vi "VelocityTorqueCurrentFOC SetControl.vi"(0 "DeviceReference":T1, 1 "StopSendingOtherRequests":bool=TRUE, 2 "Velocity":dbl, 3 "Acceleration":dbl, 4 "FeedForward":dbl, 5 "Slot":i32, 6 "OverrideCoastDurNeutral":bool, 7 "error in":errorcluster, 8 "LimitForwardMotion":bool, 9 "LimitReverseMotion":bool, 10 "IgnoreHardwareLimits":bool, 11 "UseTimesync":bool, 18 "Update Frequency (Hz)":dbl=100.0) -> (20 "DeviceReference Out":T1, 27 "error out":errorcluster)   [LabVIEW 2023]
doc: "Request PID to target velocity with torque current feedforward.\nThis control mode will set the motor's velocity setpoint to the velocity specified by the user. In addition, it will apply an additional torque current as an arbitrary feedforward value."
uses:
  Users/test.DESKTOP-CORY/Documents/PhoenixProLabVIEWGeneration/CopyDown/DeviceReference.ctl
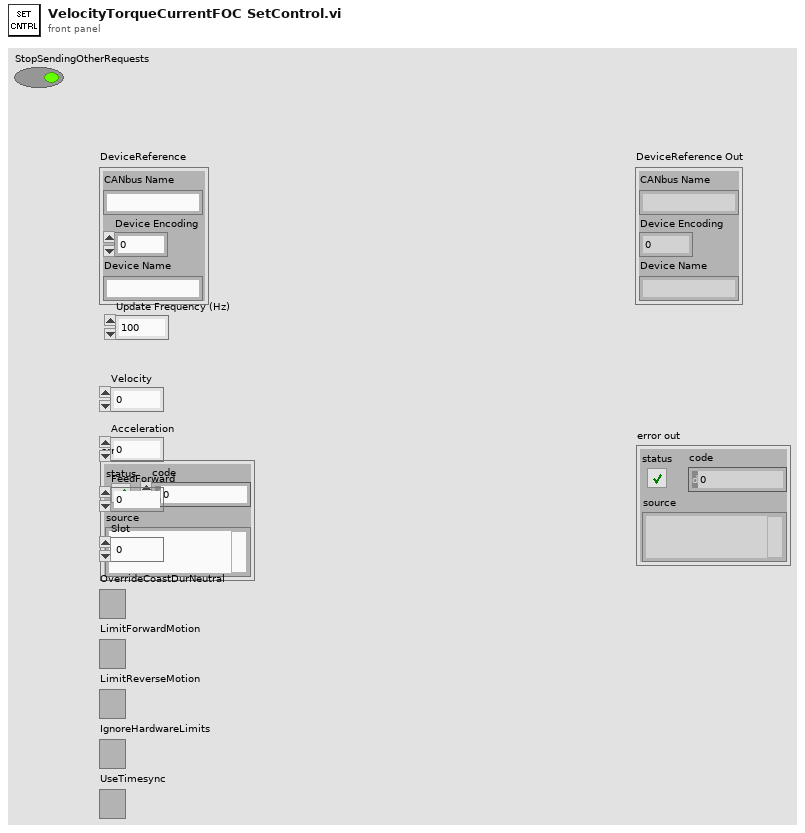
[diagram p1: front panel]
types:
  T1 = typedef "DeviceReference.ctl" = cluster{"CANbus Name":string, "Device Encoding":u32, "Device Name":string}
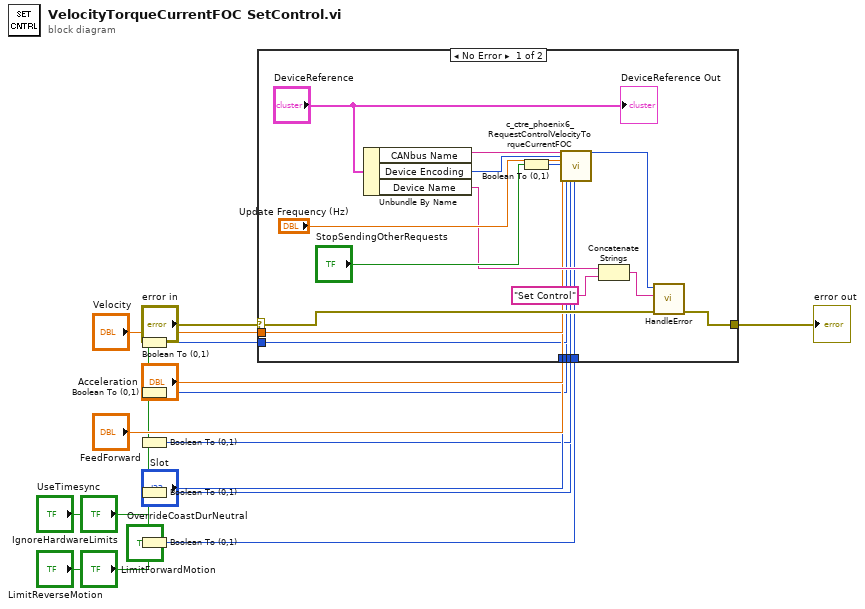
[diagram p0: block diagram]
diagram:
  n1 = Boolean To (0,1)(Boolean="OverrideCoastDurNeutral") -> (0, 1=w9:i16)
  n2 = Boolean To (0,1)(Boolean="LimitForwardMotion") -> (0, 1=w7:i16)
  n3 = Boolean To (0,1)(Boolean="LimitReverseMotion") -> (0, 1=w5:i16)
  n4 = Boolean To (0,1)(Boolean="IgnoreHardwareLimits") -> (0, 1=w3:i16)
  n5 = Boolean To (0,1)(Boolean="UseTimesync") -> (0, 1=w1:i16)
  n6 = case shown="No Error" "error in" {
    selector: "error in" -> [w30 w38]
    tunnel: [w29 w38] -> w15
    tunnel: "Velocity" -> [w25 _]
    tunnel: "Acceleration" -> [w24 _]
    tunnel: "FeedForward" -> [w23 _]
    tunnel: "Slot" -> [w22 _]
    tunnel: w9 -> [w21 _]
    tunnel: w7 -> [w20 _]
    tunnel: w5 -> [w19 _]
    tunnel: w3 -> [w18 _]
    tunnel: w1 -> [w17 _]
    frame No Error {
      n7 = Unbundle By Name("DeviceReference") -> ("CANbus Name"=w36:string, "Device Encoding"=w35:u32, "Device Name"=w28:string)
      n8 = Boolean To (0,1)(Boolean="StopSendingOtherRequests") -> (0, 1=w32:i16)
      n9 = call <vilib>:"c_ctre_phoenix6_RequestControlVelocityTorqueCurrentFOC.vi"("String 2"=w36, "Numeric 2"=w35, "Numeric 3"="Update Frequency (Hz)", "Numeric 4"=w32, "Numeric 5"=w25, "Numeric 6"=w24, "Numeric 7"=w23, "Numeric 8"=w22, "Numeric 9"=w21, "Numeric 10"=w20, "Numeric 11"=w19, "Numeric 12"=w18, 12:w17) -> ("Numeric"=w31:i32)  [unwired: 13 in, 1 out]
      n10 = Concatenate Strings(w28, "Set Control" ("origin")) -> (w26:string)
      n11 = call "HandleError.vi"("error in"=w30, "origin"=w26, "Status"=w31) -> ("error out"=w29:errorcluster)  [unwired: 8 in]
      "DeviceReference Out" <- "DeviceReference"
    }
    frame Error {
    }
  }
  "error out" <- w15
